vi "mediaIntesecaoCameras_v2.vi"(6 "grsim?":bool, 8 "cameras array":dbl[](array[numeric]), 10 "Field Geometry In":T1, 11 "Cameras Array":T2[](array[typedef]) {"robots_blue"."height" format="%+4.3f"; "robots_blue"."pixel_y" format="%+4.3f"; "robots_blue"."pixel_x" format="%+4.3f"; "robots_blue"."orientation" format="%+4.3f"; "robots_blue"."y" format="%+4.3f"; "robots_blue"."confidence" format="%4.3f"; "robots_blue"."x" format="%+4.3f"; "robots_yellow"."height" format="%+4.3f"; "robots_yellow"."pixel_y" format="%+4.3f"; "robots_yellow"."pixel_x" format="%+4.3f"; "robots_yellow"."orientation" format="%+4.3f"; "robots_yellow"."y" format="%+4.3f"; "robots_yellow"."confidence" format="%4.3f"; "robots_yellow"."x" format="%+4.3f"}) -> (3 "frame out":T2 {"robots_blue"."height" format="%+4.3f"; "robots_blue"."pixel_y" format="%+4.3f"; "robots_blue"."pixel_x" format="%+4.3f"; "robots_blue"."orientation" format="%+4.3f"; "robots_blue"."y" format="%+4.3f"; "robots_blue"."confidence" format="%4.3f"; "robots_blue"."x" format="%+4.3f"; "robots_yellow"."height" format="%+4.3f"; "robots_yellow"."pixel_y" format="%+4.3f"; "robots_yellow"."pixel_x" format="%+4.3f"; "robots_yellow"."orientation" format="%+4.3f"; "robots_yellow"."y" format="%+4.3f"; "robots_yellow"."confidence" format="%4.3f"; "robots_yellow"."x" format="%+4.3f"})   [LabVIEW 2022 SP3]
uses:
  Controls/SSL Detection Frame.ctl
  Controls/SSL Detection Robot.ctl
  <vilib>/Analysis/Matrix/Datatypes/RealMatrix.ctl
  Controls/SSL Detection Ball.ctl
  <vilib>/Analysis/Matrix/NI_Matrix.lvlib
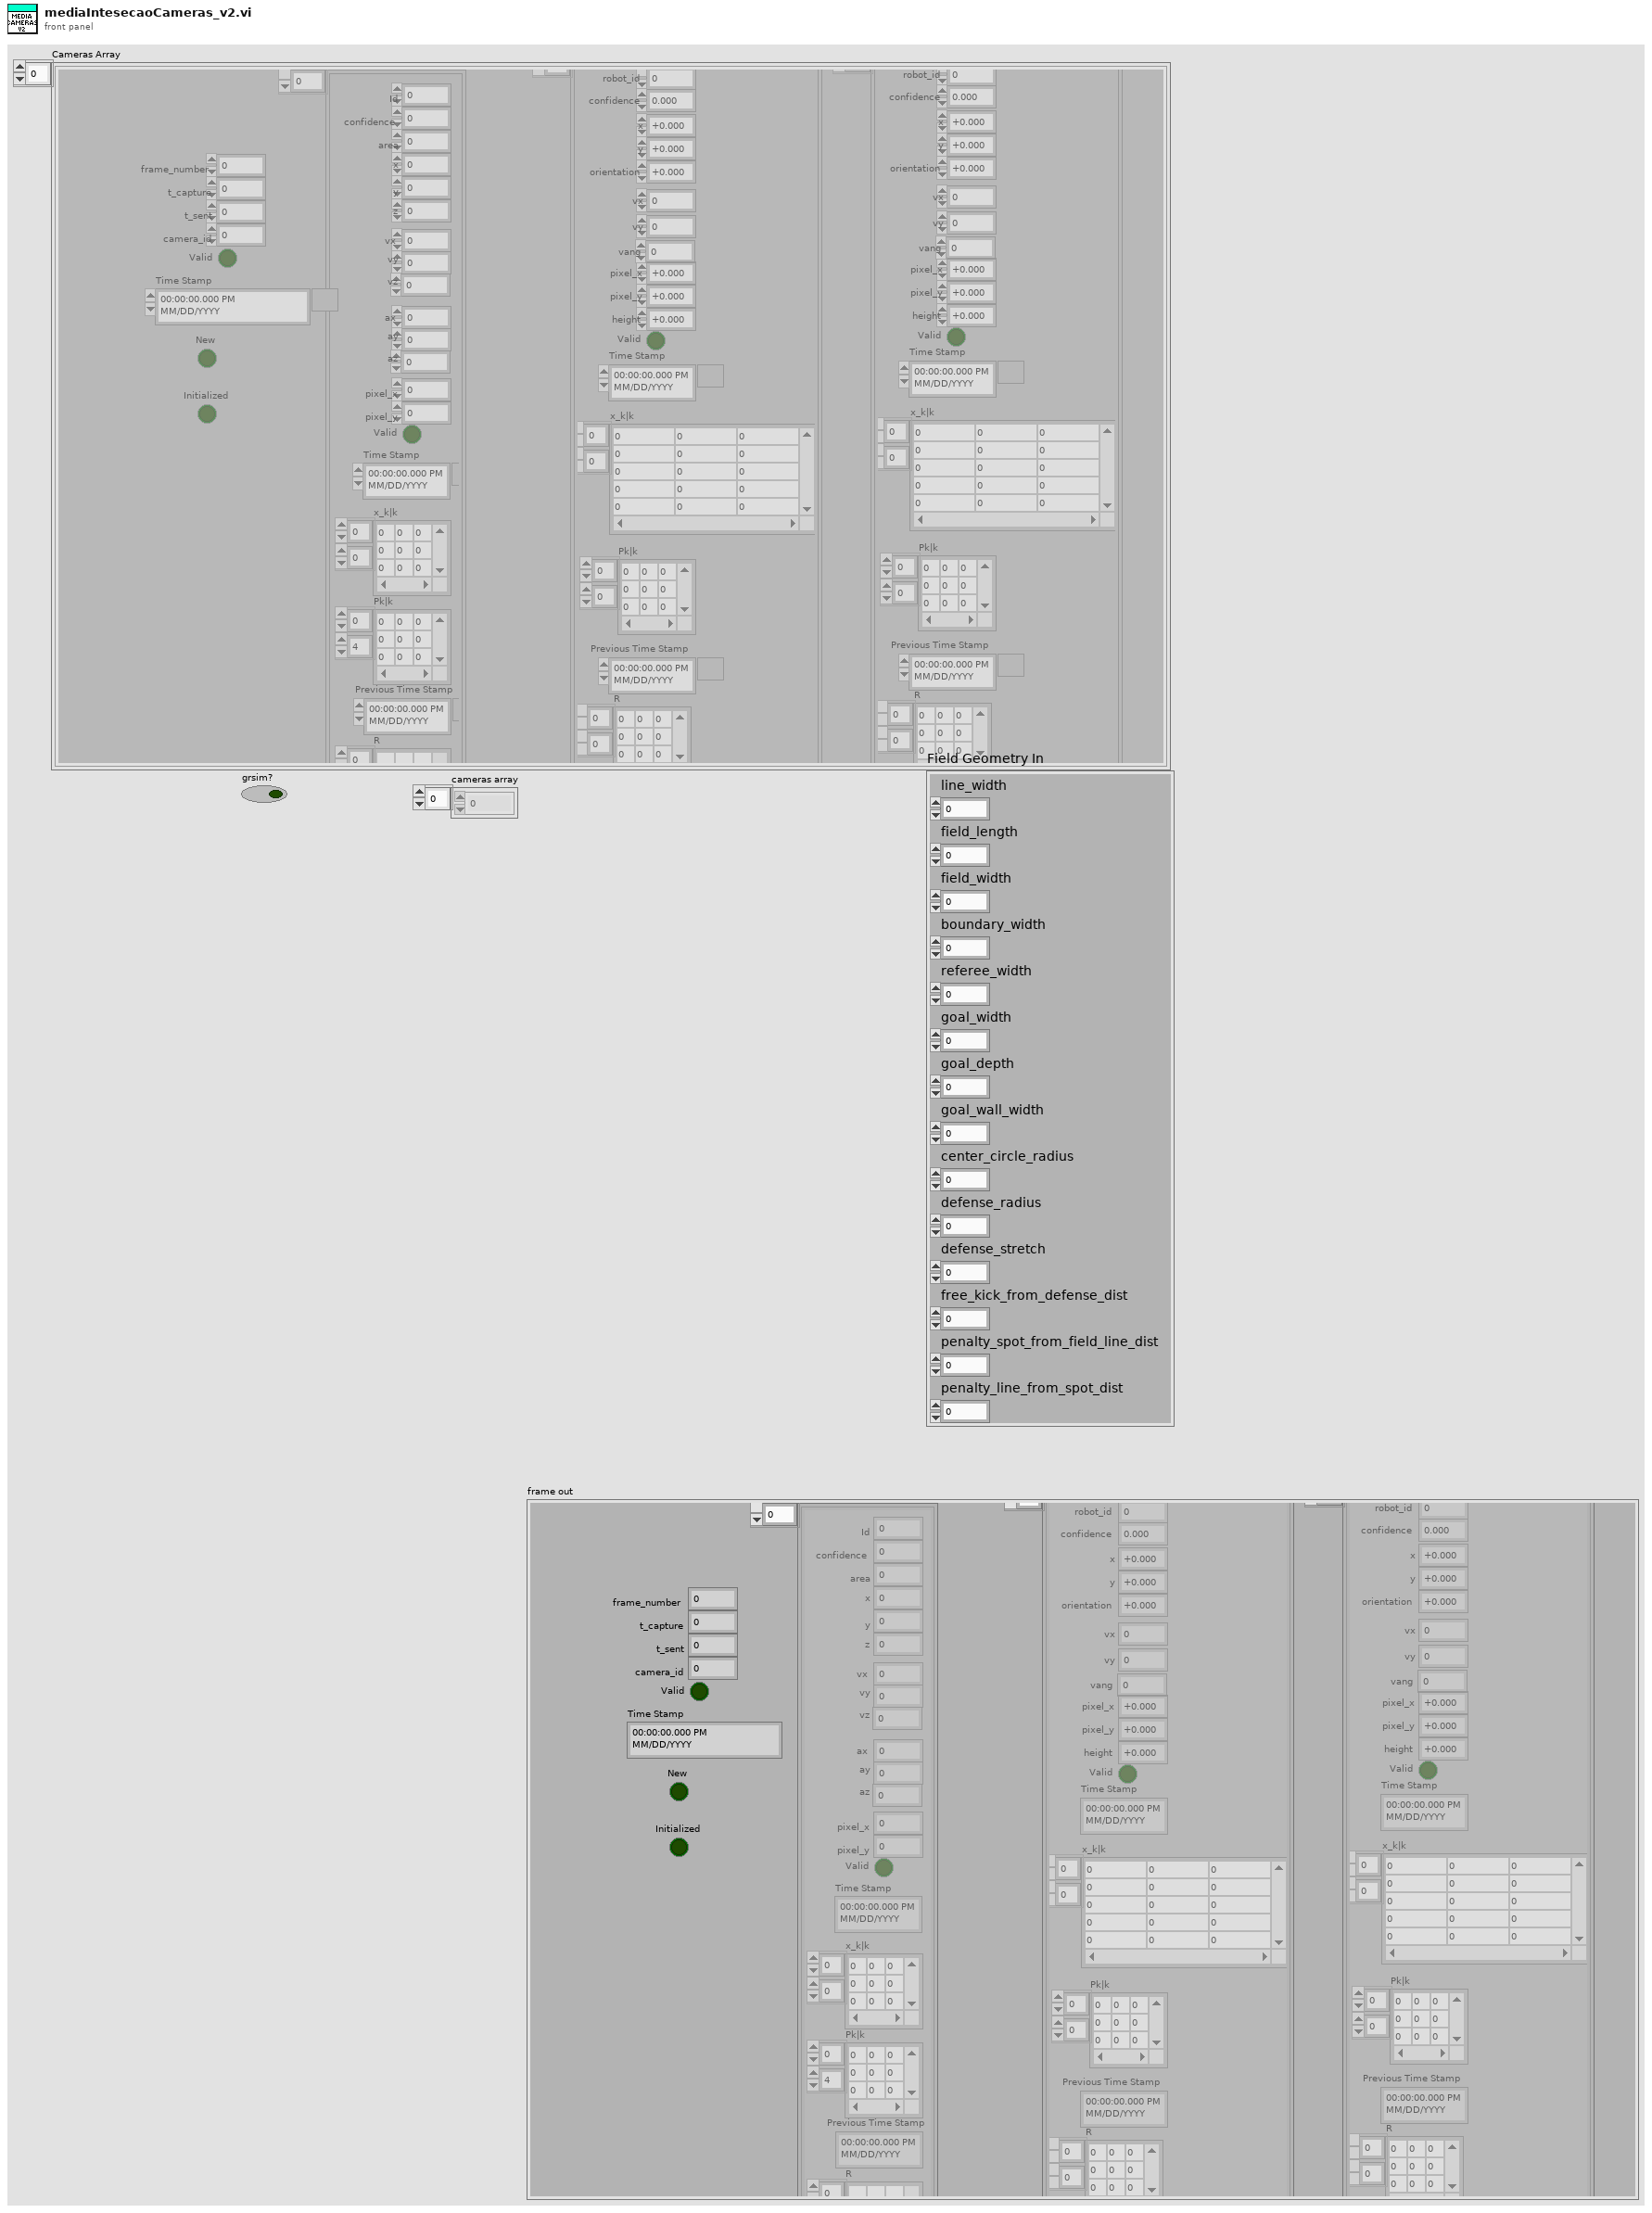
[diagram p1: front panel]
types:
  T1 = cluster{"line_width":u32, "field_length":u32, "field_width":u32, "boundary_width":u32, "referee_width":u32, "goal_width":u32, "goal_depth":u32, "goal_wall_width":u32, "center_circle_radius":u32, "defense_radius":u32, "defense_stretch":u32, "free_kick_from_defense_dist":u32, "penalty_spot_from_field_line_dist":u32, "penalty_line_from_spot_dist":u32}
  T2 = typedef "SSL Detection Frame.ctl" = cluster{"frame_number":u32, "t_capture":dbl, "t_sent":dbl, "camera_id":u32, "robots_yellow":T3[], "robots_blue":T3[], "balls":T5[], "Valid":bool, "Time Stamp":timestamp, "New":bool, "Initialized":bool}
  T3 = typedef "SSL Detection Robot.ctl" = cluster{"x":sgl, "robot_id":u32, "confidence":sgl, "y":sgl, "orientation":sgl, "pixel_x":sgl, "pixel_y":sgl, "height":sgl, "Valid":bool, "Time Stamp":timestamp, "x_k|k":T4, "Pk|k":T4, "Previous Time Stamp":timestamp, "R":T4, "vx":dbl, "vy":dbl, "vang":dbl}
  T4 = typedef "NI_Matrix.lvlib/RealMatrix.ctl" = dbl[][]
  T5 = typedef "SSL Detection Ball.ctl" = cluster{"x":sgl, "area":u32, "confidence":sgl, "y":sgl, "z":sgl, "pixel_x":sgl, "pixel_y":sgl, "Valid":bool, "Time Stamp":timestamp, "x_k|k":T4, "Pk|k":T4, "Id":u32, "Previous Time Stamp":timestamp, "R":T4, " vx":sgl, "vy":dbl, "vz":dbl, " ax":sgl, "ay":dbl, "az":dbl}
  T6 = cluster{"x":sgl, "y":sgl, "camera_id":u32, "Valid":bool}
  T7 = cluster{"x":sgl, "y":sgl, "orientation":sgl, "robot_id":u32, "camera_id":u32, "Valid":bool}
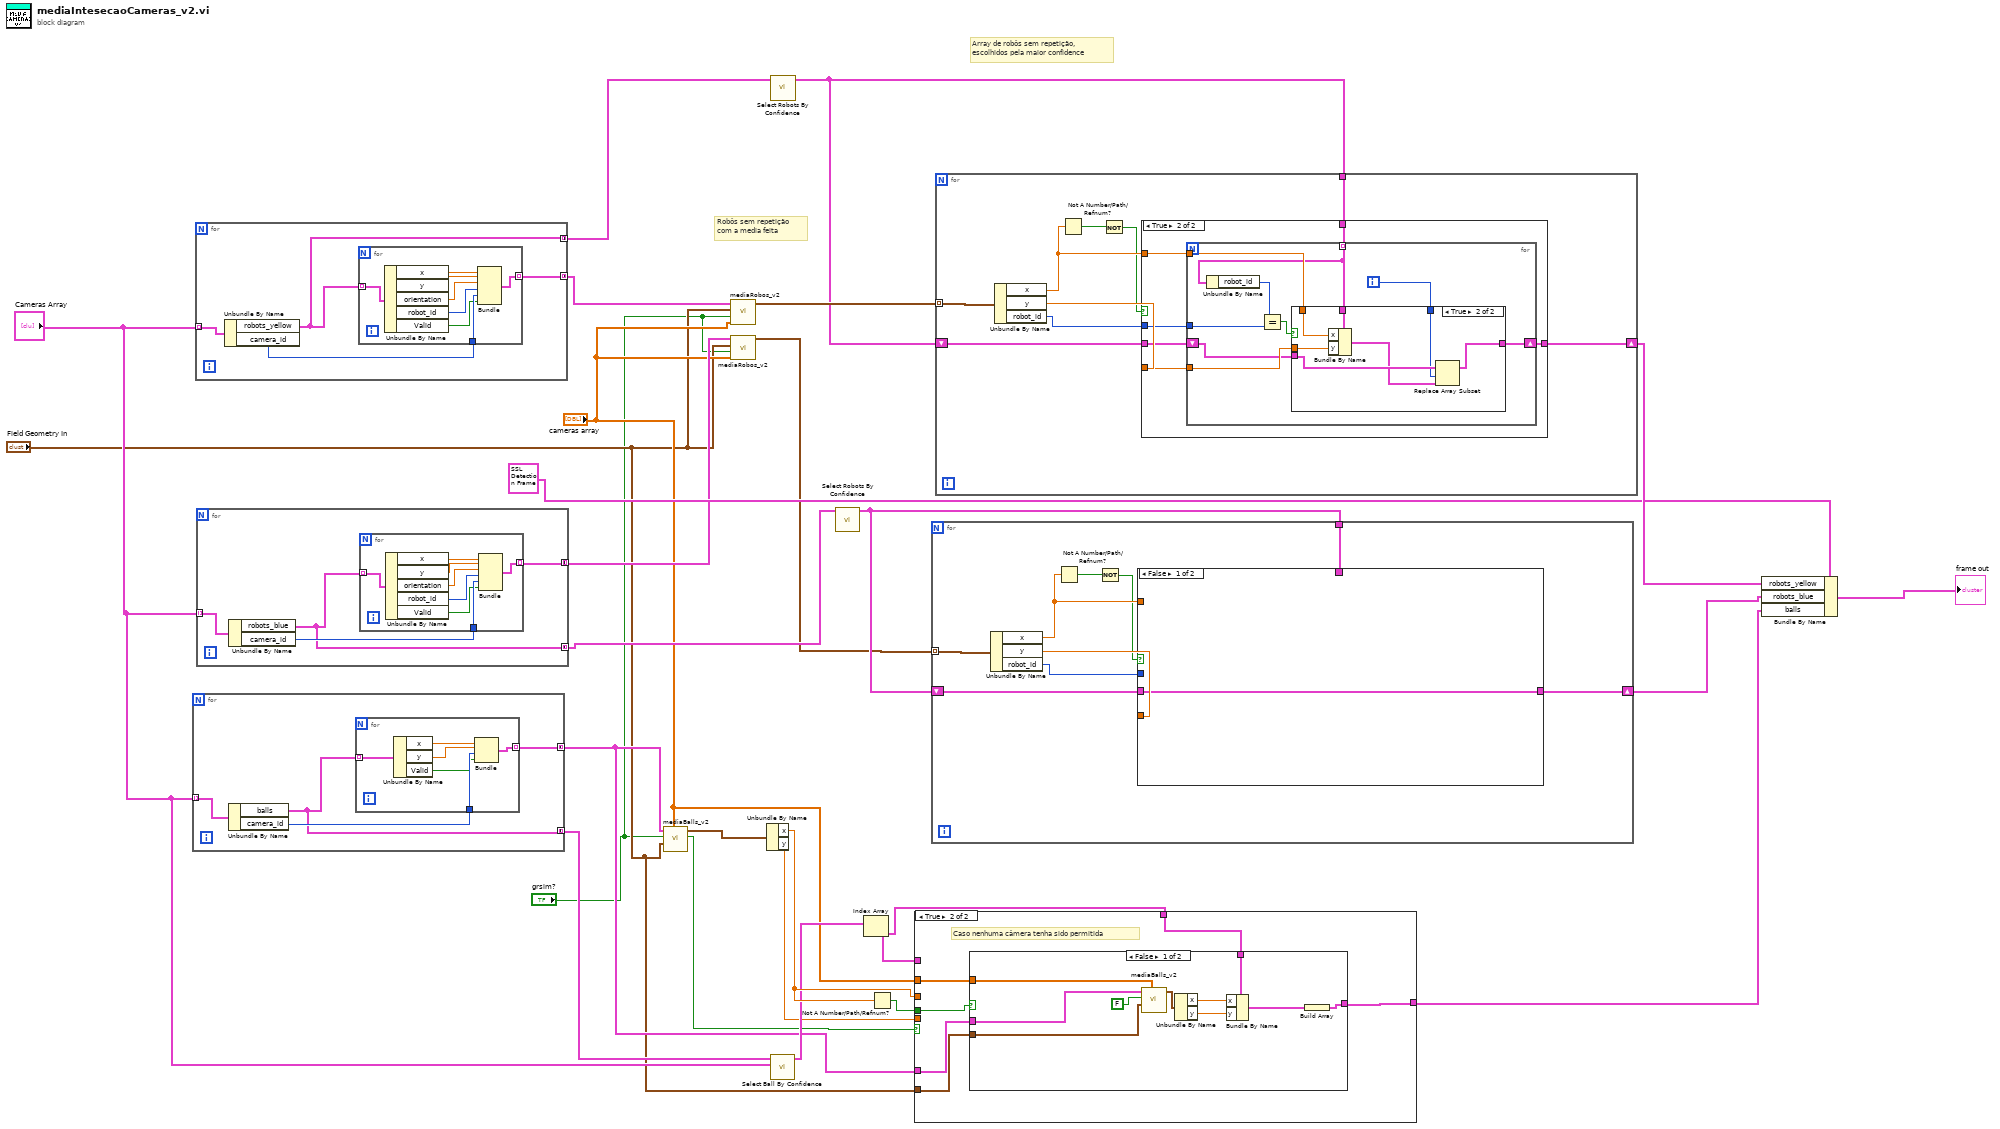
[diagram p0: block diagram]
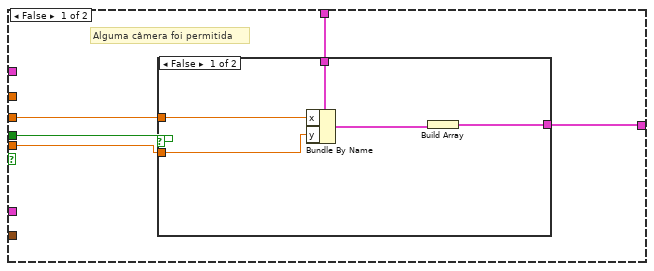
[diagram p2: hidden frame]
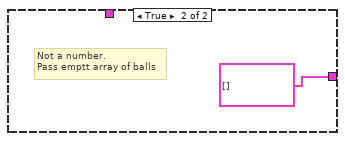
[diagram p3: hidden frame]
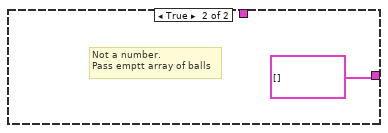
[diagram p4: hidden frame]
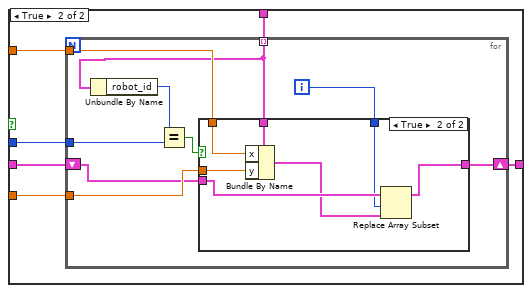
[diagram p5: hidden frame]
diagram:
  # "Robôs sem repetição \ncom a media feita"
  # "Array de robôs sem repetição,\nescolhidos pela maior confidence"
  n1 = for {
    tunnel: "Cameras Array" -> [w30] mode=indexing
    tunnel: [w29] -> w8 mode=concatenating
    tunnel: [w27] -> w17 mode=concatenating
    n2 = Unbundle By Name(w30) -> ("balls"=w27:T5[], "camera_id"=w28:u32)
    n3 = for {
      tunnel: w27 -> [w36] mode=indexing
      tunnel: [w33] -> w29 mode=indexing
      tunnel: w28 -> [w32]
      n4 = Unbundle By Name(w36) -> ("x"=w35:sgl, "y"=w34:sgl, "Valid"=w31:bool)
      n5 = Bundle("x"=w35, "y"=w34, "camera_id"=w32, "Valid"=w31) -> (w33:T6)  [unwired: 1 in]
    }
  }
  n6 = for {
    tunnel: "Cameras Array" -> [w40] mode=indexing
    tunnel: [w39] -> w10 mode=concatenating
    tunnel: [w37] -> w23 mode=concatenating
    n7 = Unbundle By Name(w40) -> ("robots_yellow"=w37:T3[], "camera_id"=w38:u32)
    n8 = for {
      tunnel: w37 -> [w48] mode=indexing
      tunnel: [w45] -> w39 mode=indexing
      tunnel: w38 -> [w42]
      n9 = Unbundle By Name(w48) -> ("x"=w47:sgl, "y"=w46:sgl, "orientation"=w44:sgl, "robot_id"=w43:u32, "Valid"=w41:bool)
      n10 = Bundle("x"=w47, "y"=w46, "orientation"=w44, "robot_id"=w43, "camera_id"=w42, "Valid"=w41) -> (w45:T7)  [unwired: 1 in]
    }
  }
  n11 = for {
    tunnel: "Cameras Array" -> [w52] mode=indexing
    tunnel: [w51] -> w12 mode=concatenating
    tunnel: [w49] -> w20 mode=concatenating
    n12 = Unbundle By Name(w52) -> ("robots_blue"=w49:T3[], "camera_id"=w50:u32)
    n13 = for {
      tunnel: w49 -> [w60] mode=indexing
      tunnel: [w57] -> w51 mode=indexing
      tunnel: w50 -> [w54]
      n14 = Unbundle By Name(w60) -> ("x"=w59:sgl, "y"=w58:sgl, "orientation"=w56:sgl, "robot_id"=w55:u32, "Valid"=w53:bool)
      n15 = Bundle("x"=w59, "y"=w58, "orientation"=w56, "robot_id"=w55, "camera_id"=w54, "Valid"=w53) -> (w57:T7)  [unwired: 1 in]
    }
  }
  n16 = call "mediaBalls_v2.vi"("cameras array"="cameras array", "Field Size"="Field Geometry In", "grSim?"="grsim?", "Array Ball Pose + CamID"=w8) -> ("No cameras?"=w6:bool, "Ball out"=w24:cluster{"x":dbl, "y":dbl})  [unwired: 6 in]
  n17 = call "mediaRobos_v2.vi"("cameras array"="cameras array", "grSim?"="grsim?", "Field Size 2"="Field Geometry In", "Array Robot Pose + CamID"=w10) -> ("Array"=w26:cluster{"x":dbl, "y":dbl, "robot_id":i32}[])  [unwired: 7 in]
  n18 = call "mediaRobos_v2.vi"("cameras array"="cameras array", "grSim?"="grsim?", "Field Size 2"="Field Geometry In", "Array Robot Pose + CamID"=w12) -> ("Array"=w7:cluster{"x":dbl, "y":dbl, "robot_id":i32}[])  [unwired: 7 in]
  n19 = Unbundle By Name(w24) -> ("x"=w11:dbl, "y"=w2:dbl)
  n20 = call "Select Ball By Confidence.vi"("Array"="Cameras Array", "balls"=w17) -> ("balls out"=w9:T5[])  [unwired: 9 in]
  n21 = call "Select Robots By Confidence.vi"("robots_blue"=w23) -> ("Array"=w22:T3[])  [unwired: 10 in]
  n22 = call "Select Robots By Confidence.vi"("robots_blue"=w20) -> ("Array"=w19:T3[])  [unwired: 10 in]
  n23 = Index Array(array=w9) -> (element=w15:T5)  [unwired: 1 in]
  n24 = Not A Number/Path/Refnum?(number/path/refnum=w11) -> (NaN/Path/Refnum?=w3:bool)
  n25 = case shown="True" w6 {
    tunnel: w15 -> [w65 w76]
    tunnel: [w63 w75] -> w14
    tunnel: w11 -> [w64 _]
    tunnel: w9 -> [_ _]
    tunnel: w8 -> [_ w77]
    tunnel: "cameras array" -> [_ w74]
    tunnel: "Field Geometry In" -> [_ w73]
    tunnel: w3 -> [w62 w72]
    tunnel: w2 -> [w61 _]
    frame False {
      # "Alguma câmera foi permitida"
      n26 = case shown="False" w62 {
        tunnel: w65 -> [w70 _]
        tunnel: w64 -> [w69 _]
        tunnel: [w67 T5[] []] -> w63
        tunnel: w61 -> [w66 _]
        frame False {
          n27 = Bundle By Name(cluster=w70, "x"=w69, "y"=w66) -> (w68:T5)
          n28 = Build Array(w68) -> (w67:T5[])
        }
        frame True {
          # "Not a number.\nPass emptt array of balls"
        }
      }
    }
    frame True {
      # "Caso nenhuma câmera tenha sido permitida"
      n29 = case shown="False" w72 {
        tunnel: w77 -> [w87 _]
        tunnel: w76 -> [w85 _]
        tunnel: [w80 T5[] []] -> w75
        tunnel: w74 -> [w79 _]
        tunnel: w73 -> [w78 _]
        frame False {
          n30 = call "mediaBalls_v2.vi"("cameras array"=w79, "Field Size"=w78, "grSim?"=FALSE, "Array Ball Pose + CamID"=w87) -> ("Ball out"=w84:cluster{"x":dbl, "y":dbl})  [unwired: 6 in, 1 out]
          n31 = Unbundle By Name(w84) -> ("x"=w83:dbl, "y"=w82:dbl)
          n32 = Bundle By Name(cluster=w85, "x"=w83, "y"=w82) -> (w81:T5)
          n33 = Build Array(w81) -> (w80:T5[])
        }
        frame True {
          # "Not a number.\nPass emptt array of balls"
        }
      }
    }
  }
  n34 = for {
    tunnel: w7 -> [w97] mode=indexing
    tunnel: w19 -> [w91]
    shift-right: [w95] -> w18
    shift-left: w19 -> [w89]
    n35 = Unbundle By Name(w97) -> ("x"=w94:dbl, "y"=w96:dbl, "robot_id"=w90:i32)
    n36 = Not A Number/Path/Refnum?(number/path/refnum=w94) -> (NaN/Path/Refnum?=w93:bool)
    n37 = Not(x=w93) -> (.not. x?=w92:bool)
    n38 = case shown="False" w92 {
      tunnel: w94 -> [_ w104]
      tunnel: w96 -> [_ w103]
      tunnel: [w98 w102] -> w95
      tunnel: w91 -> [_ w101]
      tunnel: w90 -> [_ w100]
      tunnel: w89 -> [w98 w99]
      frame False {
      }
      frame True {
        n39 = for {
          tunnel: w104 -> [w113]
          tunnel: w103 -> [w112]
          shift-right: [w106] -> w102
          shift-left: w99 -> [w107]
          tunnel: w101 -> [w108] mode=indexing
          tunnel: w100 -> [w110]
          i -> [w105]
          n40 = Unbundle By Name(w108) -> ("robot_id"=w111:u32)
          n41 = Equal?(x=w111, y=w110) -> (x = y?=w109:bool)
          n42 = case shown="True" w109 {
            tunnel: w113 -> [_ w121]
            tunnel: w112 -> [_ w120]
            tunnel: w108 -> [_ w119]
            tunnel: w107 -> [w114 w118]
            tunnel: [w114 w117] -> w106
            tunnel: w105 -> [_ w115]
            frame False {
            }
            frame True {
              n43 = Bundle By Name(cluster=w119, "x"=w121, "y"=w120) -> (w116:T3)
              n44 = Replace Array Subset(array=w118, new element=w116, index=w115) -> (w117:T3[])
            }
          }
        }
      }
    }
  }
  n45 = for {
    tunnel: w26 -> [w130] mode=indexing
    tunnel: w22 -> [w124]
    shift-right: [w128] -> w21
    shift-left: w22 -> [w122]
    n46 = Unbundle By Name(w130) -> ("x"=w127:dbl, "y"=w129:dbl, "robot_id"=w123:i32)
    n47 = Not A Number/Path/Refnum?(number/path/refnum=w127) -> (NaN/Path/Refnum?=w126:bool)
    n48 = Not(x=w126) -> (.not. x?=w125:bool)
    n49 = case shown="True" w125 {
      tunnel: w127 -> [_ w137]
      tunnel: w129 -> [_ w136]
      tunnel: [w131 w135] -> w128
      tunnel: w124 -> [_ w134]
      tunnel: w123 -> [_ w133]
      tunnel: w122 -> [w131 w132]
      frame False {
      }
      frame True {
        n50 = for {
          tunnel: w137 -> [w146]
          tunnel: w136 -> [w145]
          shift-right: [w139] -> w135
          shift-left: w132 -> [w140]
          tunnel: w134 -> [w141] mode=indexing
          tunnel: w133 -> [w143]
          i -> [w138]
          n51 = Unbundle By Name(w141) -> ("robot_id"=w144:u32)
          n52 = Equal?(x=w144, y=w143) -> (x = y?=w142:bool)
          n53 = case shown="True" w142 {
            tunnel: w146 -> [_ w154]
            tunnel: w145 -> [_ w153]
            tunnel: w141 -> [_ w152]
            tunnel: w140 -> [w147 w151]
            tunnel: [w147 w150] -> w139
            tunnel: w138 -> [_ w148]
            frame False {
            }
            frame True {
              n54 = Bundle By Name(cluster=w152, "x"=w154, "y"=w153) -> (w149:T3)
              n55 = Replace Array Subset(array=w151, new element=w149, index=w148) -> (w150:T3[])
            }
          }
        }
      }
    }
  }
  n56 = Bundle By Name(cluster=T2 {"frame_number"=0, "t_capture"=0.0, "t_sent"=0.0, "camera_id"=0, "robots_yellow"=[], "robots_blue"=[], "balls"=[], "Valid"=TRUE, "Time Stamp"=timestamp(0 s since 1904-01-01), "New"=FALSE, "Initialized"=FALSE} ("Unico frame"), "robots_yellow"=w21, "robots_blue"=w18, "balls"=w14) -> (→"frame out":T2)
